vi "X4 Encoder Count.vi"(4 "phase B_prev":bool, 5 "phase A":bool, 6 "phase B":bool, 7 "phase A_prev":bool, 11 "count in":i32) -> (2 "count changed?":bool, 3 "count out":i32)   [LabVIEW 2017, in "NI_Robotics Utilities.lvlib"]
uses:
  <vilib>/robotics/Utilities/NI_Robotics Utilities.lvlib
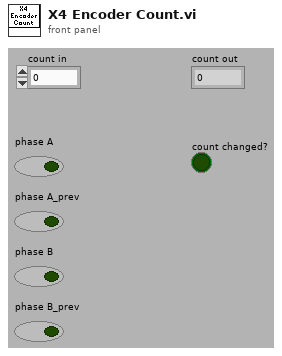
[diagram p1: front panel]
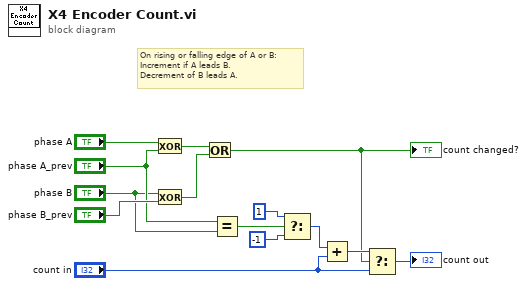
[diagram p0: block diagram]
diagram:
  # "On rising or falling edge of A or B:\nIncrement if A leads B.\nDecrement of B leads A."
  n1 = Exclusive Or(1:"phase A_prev", 2:"phase A") -> (0:w4:bool)
  n2 = Exclusive Or(1:"phase B_prev", 2:"phase B") -> (0:w5:bool)
  n3 = Or(x=w4, y=w5) -> (x .or. y?=w3:bool)
  "count changed?" <- w3
  n4 = Equal?(x="phase A_prev", y="phase B") -> (x = y?=w7:bool)
  n5 = Select(t=1 ("count in"), s=w7, f=-1 ("count in")) -> (s? t:f=w10:i32)
  n6 = Add(x=w10, y="count in") -> (x+y=w9:i32)
  n7 = Select(t=w9, s=w3, f="count in") -> (s? t:f=→"count out":i32)
